vi "wuclient.vi"() -> ()   [LabVIEW 2014]
uses:
  <vilib>/addons/zeromq/socket_type.ctl
  <vilib>/addons/zeromq/socket_options.ctl
  <vilib>/addons/zeromq/zmq_context.lvclass
  <vilib>/addons/zeromq/zeromq.lvlib
  <vilib>/addons/zeromq/zmq_socket.lvclass
panel:
  out "average temperature":dbl
  out "ITER":i32
  out "relhumidity":string
  out "temperature":string
  out "zipcode":string
  in  "iter_num":i32
  in  "FILTER":string="10001"
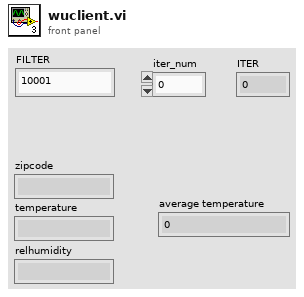
[diagram p1: front panel]
types:
  T1 = typedef "zeromq.lvlib/socket_options.ctl" = enum8{"NONE", "ZMQ_HWM", "<2>", "ZMQ_SWAP", "ZMQ_AFFINITY", "ZMQ_IDENTITY", "ZMQ_SUBSCRIBE", "ZMQ_UNSUBSCRIBE", "ZMQ_RATE", "ZMQ_RECOVERY_IVL", "ZMQ_MCAST_LOOP", "ZMQ_SNDBUF", "ZMQ_RCVBUF", "ZMQ_RCVMORE", "ZMQ_FD", "ZMQ_EVENTS", "ZMQ_TYPE", "ZMQ_LINGER", "ZMQ_RECONNECT_IVL", "ZMQ_BACKLOG", "ZMQ_RECOVERY_IVL_MSEC", "ZMQ_RECONNECT_IVL_MAX", "ZMQ_MAXMSGSIZE", "ZMQ_SNDHWM", "ZMQ_RCVHWM", "ZMQ_MULTICAST_HOPS", "<26>", "ZMQ_RCVTIMEO", "ZMQ_SNDTIMEO", "<29>", "<30>", "ZMQ_IPV4ONLY", "ZMQ_LAST_ENDPOINT", "ZMQ_ROUTER_MANDATORY", "ZMQ_TCP_KEEPALIVE", "ZMQ_TCP_KEEPALIVE_CNT", "ZMQ_TCP_KEEPALIVE_IDLE", "ZMQ_TCP_KEEPALIVE_INTVL", "ZMQ_TCP_ACCEPT_FILTER", "ZMQ_DELAY_ATTACH_ON_CONNECT", "ZMQ_XPUB_VERBOSE"}
  T2 = typedef "zeromq.lvlib/socket_type.ctl" = enum8{"ZMQ_PAIR", "ZMQ_PUB", "ZMQ_SUB", "ZMQ_REQ", "ZMQ_REP", "ZMQ_DEALER", "ZMQ_ROUTER", "ZMQ_PULL", "ZMQ_PUSH", "ZMQ_XPUB", "ZMQ_XSUB"}
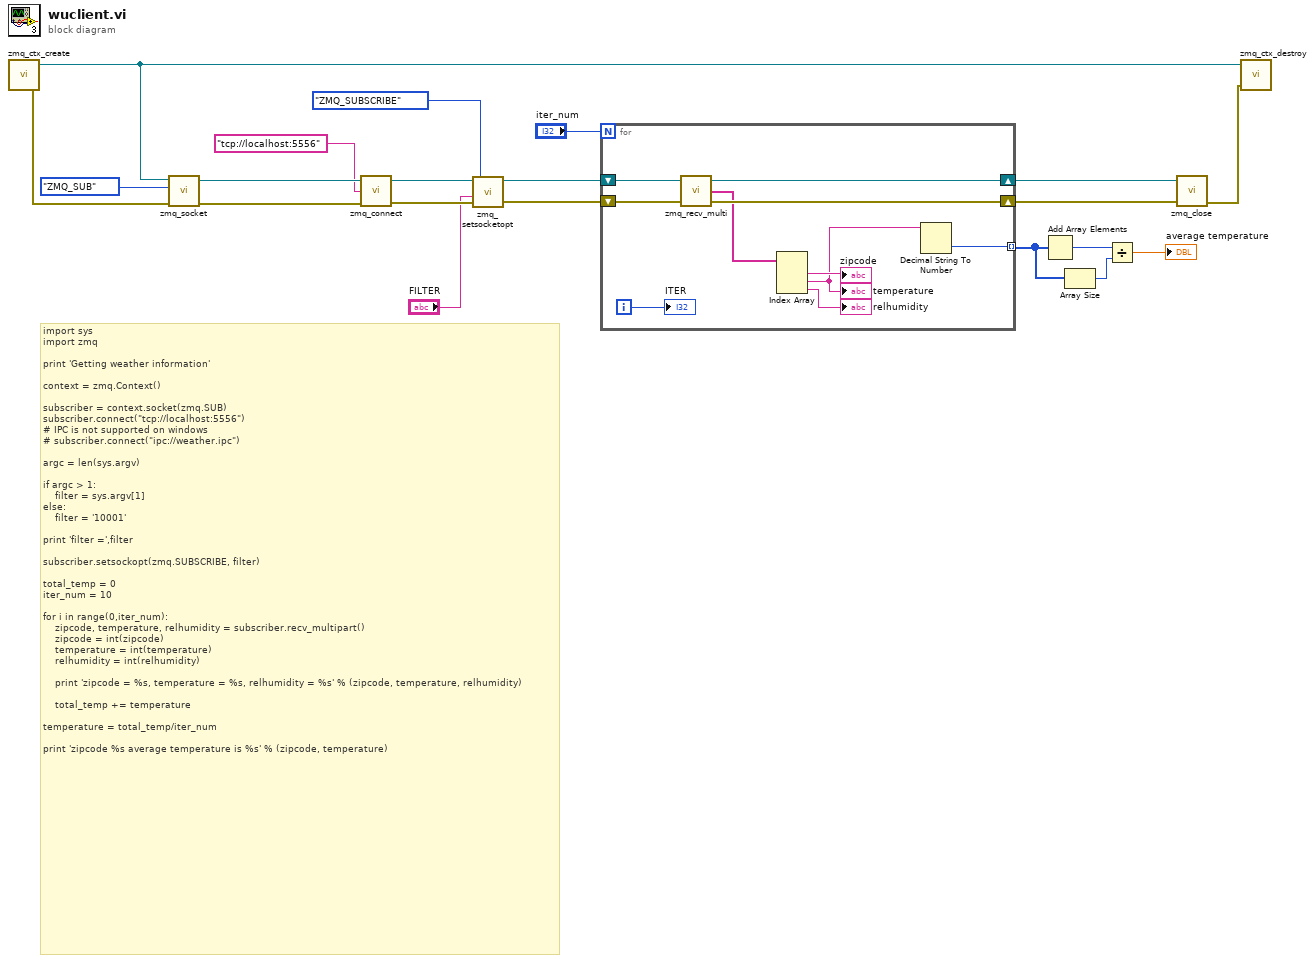
[diagram p0: block diagram]
diagram:
  # "import sys\nimport zmq\n\nprint 'Getting weather information'\n\ncontext = zmq.Context()\n\nsubscriber = context.socket(zmq.SUB)\nsubscriber.connect(\"tcp://localhost:5556\")\n# IPC is not supported on windows\n# subscriber.connect(\"ipc://weather.ipc\")\n\nargc = len(sys.argv)\n\nif argc > 1:\n    filter = sys.argv[1]\nelse:\n    filter = '10001'\n\nprint 'filter =',filter\n\nsubscriber.setsockopt(zmq.SUBSCRIBE, filter)\n\ntotal_temp = 0\niter_num = 10\n\nfor i in range(0,iter_num):\n    zipcode, temperature, relhumidity = subscriber.recv_multipart()\n    zipcode = int(zipcode)\n    temperature = int(temperature)\n    relhumidity = int(relhumidity)\n\n    print 'zipcode = %s, temperature = %s, relhumidity = %s' % (zipcode, temperature, relhumidity)\n\n    total_temp += temperature\n\ntemperature = total_temp/iter_num\n\nprint 'zipcode %s average temperature is %s' % (zipcode, temperature)"
  n1 = call <vilib>:"zmq_ctx_create.vi"() -> ("error out"=w19:errorcluster, "context out"=w18:refnum<class "zmq_context.lvclass">)  [unwired: 4 in]
  n2 = call <vilib>:"zmq_socket.vi"("error in"=w19, "socket type"=socket_type."ZMQ_SUB", "context in"=w18) -> ("error out"=w16:errorcluster, "socket out"=w17:refnum<class "zmq_socket.lvclass">)  [unwired: 2 in, 1 out]
  n3 = call <vilib>:"zmq_connect.vi"("error in"=w16, "endpoint"="tcp://localhost:5556", "socket in"=w17) -> ("error out"=w9:errorcluster, "socket out"=w11:refnum<class "zmq_socket.lvclass">)  [unwired: 1 in]
  n4 = call <vilib>:"zmq_setsocketopt.vi"("error in"=w9, "value"="FILTER", "option"=socket_options."ZMQ_SUBSCRIBE", "socket in"=w11) -> ("error out"=w8:errorcluster, "socket out"=w10:refnum<class "zmq_socket.lvclass">)  [unwired: 2 in]
  n5 = for {
    N: "iter_num" -> [_]
    shift-right: [w30] -> w13
    shift-left: w10 -> [w28]
    shift-right: [w29] -> w12
    shift-left: w8 -> [w27]
    tunnel: [w21] -> w2 mode=indexing
    i -> [w26]
    n6 = call <vilib>:"zmq_recv_multi.vi"("error in"=w27, "socket in"=w28) -> ("error out"=w29:errorcluster, "parts"=w25:string[], "socket out"=w30:refnum<class "zmq_socket.lvclass">)  [unwired: 1 in]
    n7 = Index Array(array=w25) -> (element #1=→"zipcode":string, element #2=w22:string, element #3=→"relhumidity":string)  [unwired: 3 in]
    "temperature" <- w22
    n8 = Decimal String To Number(string=w22) -> (number=w21:i32)  [unwired: 2 in, 1 out]
    "ITER" <- w26
  }
  n9 = Add Array Elements(numeric array=w2) -> (sum=w4:i32)
  n10 = Array Size(array=w2) -> (size(s)=w3:i32)
  n11 = Divide(x=w4, y=w3) -> (x/y=→"average temperature":dbl)
  n12 = call <vilib>:"zmq_close.vi"("error in"=w12, "socket"=w13) -> ("error out"=w14:errorcluster)  [unwired: 3 in]
  n13 = call <vilib>:"zmq_ctx_destroy.vi"("error in"=w14, "context in"=w18) -> ()  [unwired: 3 in, 1 out]
